vi "Globals.vi"() -> ()   [LabVIEW 2017]
panel:
  in  "Stop SubPanel":refnum<user-event>
  in  "SubPanel Event":refnum<user-event>
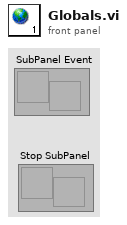
[diagram p1: front panel]
diagram:
